vi "loadDataToBuffer.vi"(8 "error in (no error)":errorcluster, 11 "niDAQmxDO in":refnum<class "niDAQmxDO.lvclass">) -> (0 "error out":errorcluster, 3 "niDAQmxDO out":refnum<class "niDAQmxDO.lvclass">)   [LabVIEW 2011, in "Hardware.lvlib" / "Channels.lvlib" / "niDAQmxDO.lvclass"]
uses:
  niDAQmxDO.lvclass
  <vilib>/DAQmx/write.llb/DAQmx Write (Digital 1D Wfm NChan NSamp).vi
  <vilib>/Waveform/DWDTOps.llb/DWDT Uncompress Digital.vi
  <vilib>/DAQmx/miscellaneous.llb/DAQmx Fill In Error Info.vi
  Program Files/National Instruments/LabVIEW 2011/resource/objmgr/daqmx.rc
panel:
  out "TotalNumber of sample per channel":i32
  out "number of samples written per channel":u32
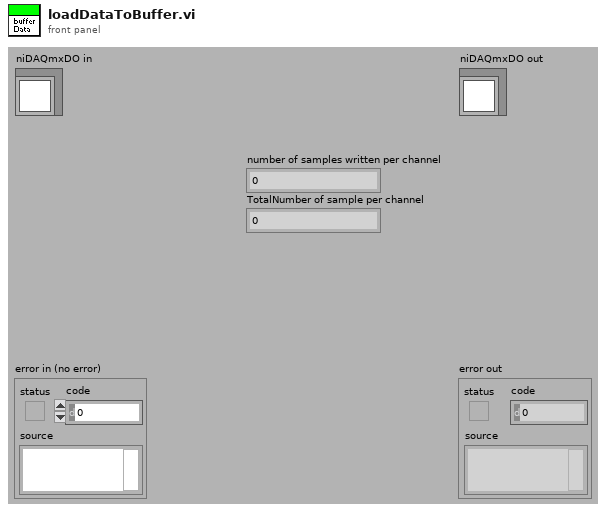
[diagram p1: front panel]
types:
  T1 = cluster{"Timestamps ms":dbl[], "DataPerChannel":dbl[][]}
  T2 = cluster{"Timestamps ms":dbl[], "Bitmap":bool[][]}
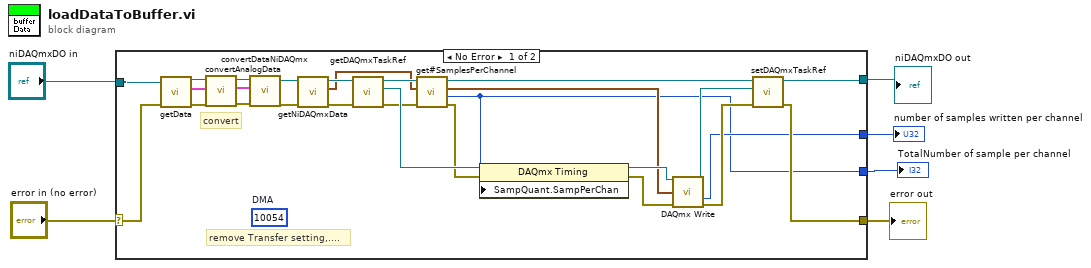
[diagram p0: block diagram]
diagram:
  n1 = case shown="No Error" "error in (no error)" {
    selector: "error in (no error)" -> [w32 w34]
    tunnel: [w28 w35] -> w4
    tunnel: "niDAQmxDO in" -> [w33 w35]
    tunnel: [w29 w34] -> w3
    tunnel: [w14 _] -> w2
    tunnel: [w7 _] -> w1
    frame No Error {
      (unwired) 10054  # DMA
      # "remove Transfer setting,...."
      # "convert"
      n2 = call-dynamic "getData.vi"("error in (no error)"=w32, "DigitalOutput.lvclass in"=w33) -> ("error out"=w19:errorcluster, "Data"=w20:T1, "DigitalOutput.lvclass out"=w21:refnum<class "niDAQmxDO.lvclass">)  [unwired: 7 in]
      n3 = call "convertAnalogData.vi"("error in (no error)"=w19, "Data"=w20, "niDAQmxDO in"=w21) -> ("error out"=w18:errorcluster, "digitalData"=w22:T2, "niDAQmxDO out"=w23:refnum<class "niDAQmxDO.lvclass">)  [unwired: 6 in]
      n4 = call "convertDataNiDAQmx.vi"("error in (no error)"=w18, "Data"=w22, "niDAQmxDO in"=w23) -> ("error out"=w26:errorcluster, "niDAQmxDO out"=w27:refnum<class "niDAQmxDO.lvclass">)  [unwired: 7 in]
      n5 = call "getNiDAQmxData.vi"("error in (no error)"=w26, "niDAQmxDO.lvclass in"=w27) -> ("error out"=w24:errorcluster, "NIDAQmx data format"=w12:digitalwaveform[], "niDAQmxDO.lvclass out"=w25:refnum<class "niDAQmxDO.lvclass">)  [unwired: 7 in]
      n6 = call "getDAQmxTaskRef.vi"("error in (no error)"=w24, "niDAQmxDO.lvclass in"=w25) -> ("error out"=w11:errorcluster, "DAQmx Task Ref"=w17:refnum<k21>, "niDAQmxDO.lvclass out"=w13:refnum<class "niDAQmxDO.lvclass">)  [unwired: 7 in]
      n7 = call "get#SamplesPerChannel.vi"("error in (no error)"=w11, "NIDAQmx data format"=w12, "niDAQmxDO in"=w13) -> ("error out"=w8:errorcluster, "samplesPerChannel"=w7:i32, "NIDAQmx data format out"=w10:digitalwaveform[], "niDAQmxDO out"=w9:refnum<class "niDAQmxDO.lvclass">)  [unwired: 5 in]
      n8 = property class="DAQmx Timing"(reference=w17, error in=w8, "SampQuant.SampPerChan"=w7) -> (reference out=w15:refnum<k21>, error out=w16:errorcluster)
      n9 = call-poly <vilib>:"DAQmx Write.vi"("task/channels in"=w15, "data"=w10, "error in"=w16) -> ("task out"=w30:refnum<k21>, "number of samples written per channel"=w14:u32, "error out"=w31:errorcluster)  [unwired: 10 in]
      n10 = call "setDAQmxTaskRef.vi"("error in (no error)"=w31, "DAQmx Task Ref"=w30, "niDAQmxDO.lvclass in"=w9) -> ("error out"=w29:errorcluster, "niDAQmxDO.lvclass out"=w28:refnum<class "niDAQmxDO.lvclass">)  [unwired: 7 in]
    }
    frame Error {
    }
  }
  "error out" <- w3
  "niDAQmxDO out" <- w4
  "number of samples written per channel" <- w2
  "TotalNumber of sample per channel" <- w1
